vi "drive-spin-sim.vi"(11 "Motor Demand":dbl) -> (3 "Rotation Change Deg":dbl)   [LabVIEW 2019]
uses:
  <vilib>/ptbypt/NI_PtbyPt.lvlib
  <vilib>/Rock Robotics/WPI/ThirdParty/JAS_Junk/TrajLib/Trajectory_Library.lvlib
  <vilib>/Rock Robotics/WPI/ThirdParty/JAS_Junk/TrajLib/LinearFilter_LP_BW1_Execute.vi
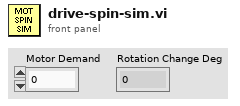
[diagram p1: front panel]
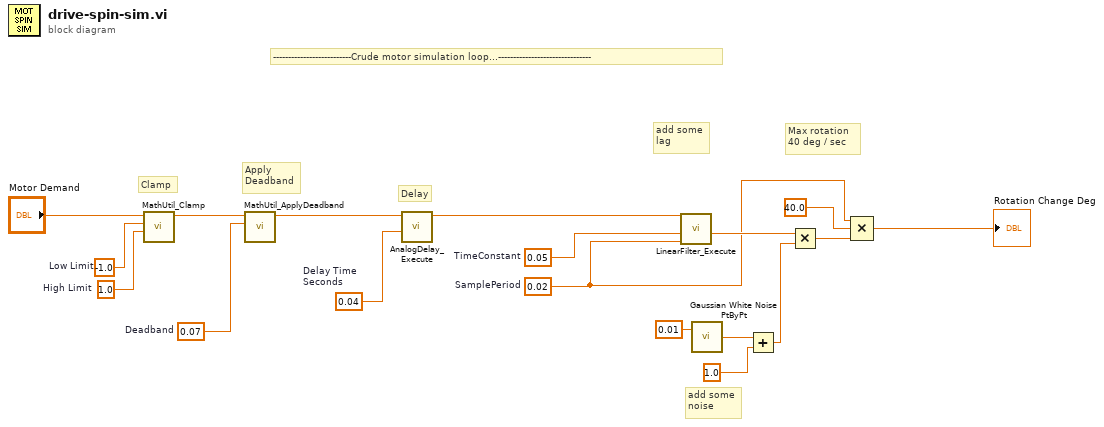
[diagram p0: block diagram]
diagram:
  w4 = 0.07  # Deadband
  w6 = 0.04  # Delay Time Seconds
  w10 = 1.0  # High Limit
  w9 = -1.0  # Low Limit
  w7 = 0.02  # SamplePeriod
  w1 = 0.05  # TimeConstant
  # "Apply\nDeadband"
  # "Delay"
  # "Max rotation \n40 deg / sec"
  # "Clamp"
  # "add some\nnoise"
  # "add some\nlag"
  # "--------------------------Crude motor simulation loop...-------------------------------"
  n1 = call <vilib>:"MathUtil_Clamp.vi"("High Limit"=w10, "Low Limit"=w9, "Value"="Motor Demand") -> ("Result"=w3:dbl)  [unwired: 8 in]
  n2 = call <vilib>:"MathUtil_ApplyDeadband.vi"("Deadband"=w4, "Value"=w3) -> ("Result"=w2:dbl)  [unwired: 9 in]
  n3 = call <vilib>:"AnalogDelay_Execute.vi"("Delay Time"=w6, "Input"=w2) -> ("Output"=w5:dbl)  [unwired: 8 in, 1 out]
  n4 = call-poly <vilib>:"LinearFilter_Execute.vi"("SamplePeriod"=w7, "TimeConstant"=w1, "Input"=w5) -> ("Output"=w14:dbl)  [unwired: 8 in]
  n5 = call <vilib>:"Gaussian White Noise PtByPt.vi"("standard deviation"=0.01) -> ("Gaussian white noise"=w15:dbl)  [unwired: 2 in]
  n6 = Add(x=w15, y=1.0) -> (x+y=w13:dbl)
  n7 = Multiply(x=w14, y=w13) -> (x*y=w12:dbl)
  n8 = Compound Arithmetic op=MULTIPLY(w7, 40.0 ("value"), w12) -> (→"Rotation Change Deg":dbl)
